vi "Initialize.vi"(8 "error in (no error)":errorcluster, 9 "Reset (True)":bool=TRUE, 10 "ID Query (True)":bool=TRUE, 11 "VISA resource name":refnum<visa-resource-name>) -> (0 "error out":errorcluster, 3 "VISA resource name out":refnum<visa-resource-name>)   [LabVIEW 2015, in "Fluke 289.lvlib"]
doc: "Establishes communication with the instrument and optionally performs an instrument identification query and/or an instrument reset. It also places the instrument in a default state needed for other instrument driver operations. Therefore, call this VI before calling other instrument driver VIs for this instrument. Generally, you need to call the Initialize VI only once at the beginning of an application."
uses:
  <instrlib>/Fluke 289/Fluke 289.lvlib
panel:
  # "(c) 2014 National Instruments.  ALL RIGHTS RESERVED."
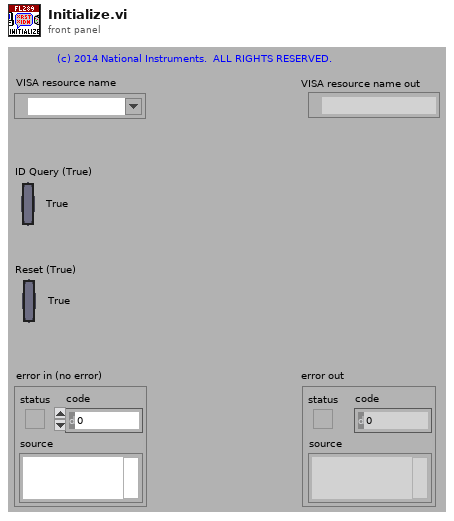
[diagram p1: front panel]
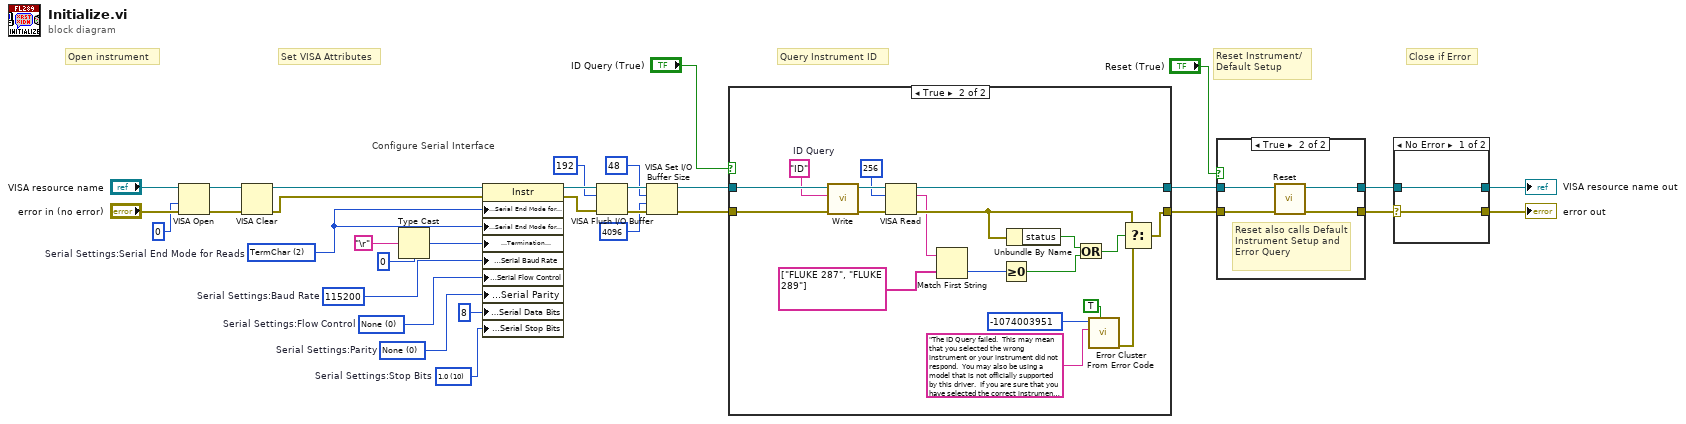
[diagram p0: block diagram]
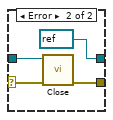
[diagram p2: hidden frame]
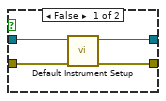
[diagram p3: hidden frame]
diagram:
  w1 = u16 0 items=["None", "XON/XOFF", "RTS/CTS", "XON/XOFF & RTS/CTS", "DTR/DSR", "XON/XOFF & DTR/DSR"]  # Serial Settings:Flow Control
  w2 = u16 0 items=["None", "Odd", "Even", "Mark", "Space"]  # Serial Settings:Parity
  w4 = u16 10 items=["1.0"=10, "1.5"=15, "2.0"=20]  # Serial Settings:Stop Bits
  w5 = u32 115200  # Serial Settings:Baud Rate
  w12 = u16 2 items=["None", "LastBit", "TermChar"]  # Serial Settings:Serial End Mode for Reads
  # "Configure Serial Interface"
  # "Set VISA Attributes"
  # "Close if Error"
  # "Query Instrument ID"
  # "Reset Instrument/\nDefault Setup"
  # "Open instrument"
  n1 = VISA Open(access mode=u32 0, error in (no error)="error in (no error)", VISA resource name="VISA resource name") -> (VISA resource name=w26:refnum<visa-resource-name>, error out=w25:errorcluster)  [unwired: 2 in]
  n2 = VISA Clear(VISA resource name=w26, error in (no error)=w25) -> (VISA resource name out=w8:refnum<visa-resource-name>, error out=w7:errorcluster)
  n3 = Type Cast(type=u8 0, x="\r") -> (*(type *) &x=w11:u8)
  n4 = property class="Instr"(reference=w8, error in=w7, "Serial Settings:Serial End Mode for Reads"=w12, "Serial Settings:Serial End Mode for Writes"=w12, "Message Based Settings:Termination Character"=w11, "Serial Settings:Serial Baud Rate"=w5, "Serial Settings:Serial Flow Control"=w1, "Serial Settings:Serial Parity"=w2, "Serial Settings:Serial Data Bits"=u16 8 ("Serial Settings:Data Bits"), "Serial Settings:Serial Stop Bits"=w4) -> (reference out=w17:refnum<visa-resource-name>, error out=w19:errorcluster)
  n5 = VISA Flush I/O Buffer(VISA resource name=w17, mask (16)=u16 192, error in (no error)=w19) -> (VISA resource name out=w20:refnum<visa-resource-name>, error out=w18:errorcluster)
  n6 = VISA Set I/O Buffer Size(VISA resource name=w20, mask (16)=u16 48, size (4096)=u32 4096 ("size (0)"), error in (no error)=w18) -> (VISA resource name out=w10:refnum<visa-resource-name>, error out=w9:errorcluster)
  n7 = case shown="True" "ID Query (True)" {
    tunnel: [w34 w54] -> w32
    tunnel: [w35 w51] -> w33
    tunnel: w10 -> [w35 w52]
    tunnel: w9 -> [w34 w53]
    frame False {
    }
    frame True {
      w47 = "ID"  # ID Query
      n8 = call <instrlib>:"Write.vi"("error in (no error)"=w53, "Write Buffer"=w47, "VISA resource name"=w52) -> ("error out"=w49:errorcluster, "VISA resource name out"=w50:refnum<visa-resource-name>)  [unwired: 7 in]
      n9 = VISA Read(VISA resource name=w50, byte count=u32 256, error in (no error)=w49) -> (VISA resource name out=w51:refnum<visa-resource-name>, read buffer=w37:string, error out=w42:errorcluster)  [unwired: 1 out]
      n10 = Match First String(2:string[] ["FLUKE 287", "FLUKE 289"], 3:w37) -> (0:w36:i32)  [unwired: 1 out]
      n11 = Greater Or Equal To 0?(x=w36) -> (x >= 0?=w40:bool)
      n12 = Unbundle By Name(w42) -> ("status"=w41:bool)
      n13 = Or(x=w41, y=w40) -> (x .or. y?=w39:bool)
      n14 = call <vilib>:"Error Cluster From Error Code.vi"("show call chain? (False)"=TRUE, "error message (\"\")"="The ID Query failed.  This may mean that you selected the wrong instrument or your instrument did not respond.  You may also be using a model that is not officially supported by this driver.  If you are sure that you have selected the correct instrument and it is responding, try disabling the ID Query." ("Source (VI Name)"), "error code (0)"=-1074003951 ("Code")) -> ("error out"=w46:errorcluster)  [unwired: 6 in]
      n15 = Select(t=w42, s=w39, f=w46) -> (s? t:f=w54:errorcluster)
    }
  }
  n16 = case shown="True" "Reset (True)" {
    tunnel: w32 -> [w57 w59]
    tunnel: [w55 w62] -> w21
    tunnel: w33 -> [w58 w60]
    tunnel: [w56 w61] -> w22
    frame False {
      n17 = call <instrlib>:"Default Instrument Setup.vi"("error in (no error)"=w57, "VISA resource name"=w58) -> ("error out"=w55:errorcluster, "VISA resource name out"=w56:refnum<visa-resource-name>)  [unwired: 8 in]
    }
    frame True {
      # "Reset also calls Default Instrument Setup and Error Query"
      n18 = call <instrlib>:"Reset.vi"("error in (no error)"=w59, "VISA resource name"=w60) -> ("error out"=w62:errorcluster, "VISA resource name out"=w61:refnum<visa-resource-name>)  [unwired: 8 in]
    }
  }
  n19 = case shown="No Error" w21 {
    selector: w21 -> [w63 w66]
    tunnel: w22 -> [w64 w67]
    tunnel: [w64 refnum<visa-resource-name> refnum ("VISA resource name out")] -> w24
    tunnel: [w63 w68] -> w23
    frame No Error {
    }
    frame Error {
      n20 = call <instrlib>:"Close.vi"("error in (no error)"=w66, "VISA resource name"=w67) -> ("error out"=w68:errorcluster)  [unwired: 9 in]
    }
  }
  "VISA resource name out" <- w24
  "error out" <- w23
